vi "get sonde data.vi"(8 "error in (no error)":errorcluster, 11 "Sonde Output File Path":path) -> (0 "error out":errorcluster, 1 "Sample Row \nBreak points":i32[](array[numeric]), 2 "Sample Array":i32[](array[numeric]), 3 "Sonde Data":string[][](array[string]))   [LabVIEW 2016]
uses:
  <vilib>/Utility/file.llb/Read Delimited Spreadsheet (string).vi
panel:
  out "Sample column":string[](array[string])
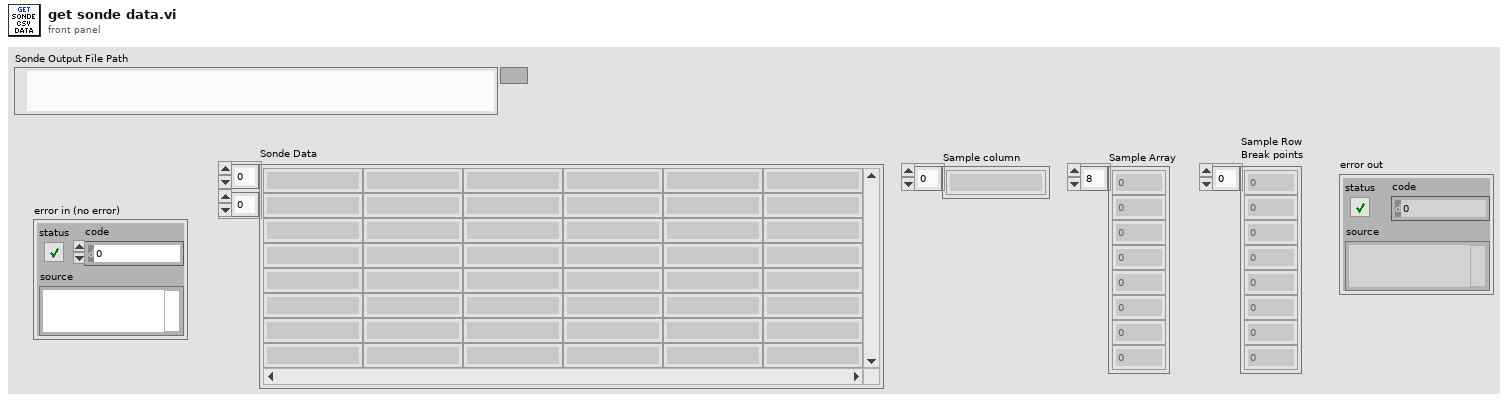
[diagram p1: front panel]
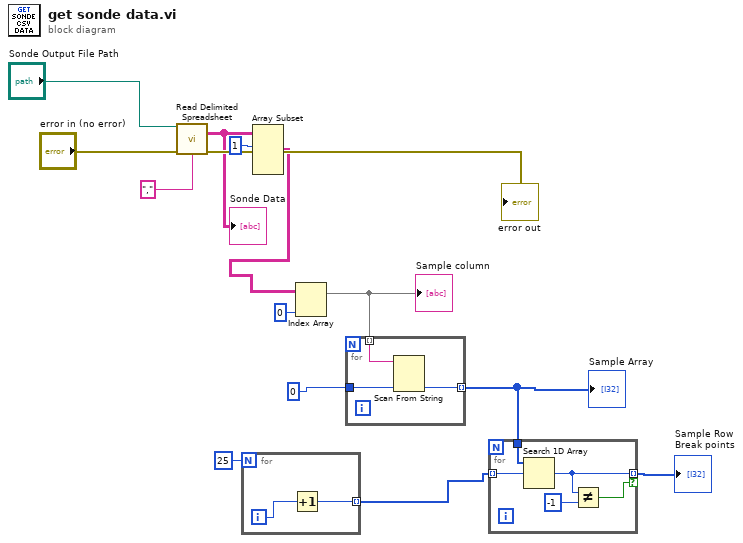
[diagram p0: block diagram]
diagram:
  n1 = call-poly <vilib>:"Read Delimited Spreadsheet.vi"("file path (dialog if empty)"="Sonde Output File Path", "error in (no error)"="error in (no error)", "delimiter (\\t)"="," ("delimiter (\\t)")) -> ("all rows"=w9:string[][], "error out"=→"error out":errorcluster)  [unwired: 7 in, 4 out]
  "Sonde Data" <- w9
  n2 = for {
    N: 25 -> [_]
    tunnel: [w15] -> w2 mode=indexing
    i -> [w16]
    n3 = Increment(x=w16) -> (x+1=w15:i32)
  }
  n4 = Array Subset(array=w9, index (row)=1 ("index")) -> (w7:string[][])  [unwired: 3 in]
  n5 = Index Array(array=w7, index (col)=0 ("disabled index (col)")) -> (element=w6:string[])  [unwired: 1 in]
  "Sample column" <- w6
  n6 = for {
    tunnel: w6 -> [w19] mode=indexing
    tunnel: 0 -> [w18]
    tunnel: [w17] -> w4 mode=indexing
    n7 = Scan From String(input string=w19, default 1=w18) -> (output 1=w17:i32)  [unwired: 3 in, 3 out]
  }
  "Sample Array" <- w4
  n8 = for {
    tunnel: w4 -> [w24]
    tunnel: w2 -> [w23] mode=indexing
    tunnel: [w22] -> w1 mode=indexing if=w20
    n9 = Search 1D Array(1D array=w24, element=w23) -> (index of element=w22:i32)  [unwired: 1 in]
    n10 = Not Equal?(x=w22, y=-1) -> (x != y?=w20:bool)
  }
  "Sample Row \nBreak points" <- w1
